vi "Entry.vi"(8 "error in (no error)":errorcluster, 11 "New State":refnum<class "Init.lvclass">) -> (0 "error out":errorcluster, 3 "State out":refnum<class "Init.lvclass">)   [LabVIEW 2024, in "Chef State.lvlib" / "Init.lvclass"]
doc: "This is an abstract method. Override this method to define the behavior when you enter the state."
uses:
  Init.lvclass
  C:/Program Files/National Instruments/LabVIEW 2024/vi.lib/ActorFramework/Actor/Actor.lvclass
  <vilib>/ActorFramework/Actor/Actor.lvclass/Actor.ctl
  Chef UI Logic/Chef UI Logic Messages/Update Log Msg/Update Log Msg.lvclass/Update Log Msg.ctl
  <vilib>/ActorFramework/Message Enqueuer/Message Enqueuer.lvclass/Message Enqueuer.ctl
  <vilib>/ActorFramework/Message Enqueuer/Enqueue.vi
  <vilib>/ActorFramework/Message Enqueuer/Init from Existing Queue.vi
  Chef UI Logic/Chef UI Logic Messages/Update Log Msg/Update Log Msg.lvclass
  C:/Program Files/National Instruments/LabVIEW 2024/vi.lib/ActorFramework/Message/Message.lvclass
  Chef State Messages/Go to Idle Msg/Go to Idle Msg.lvclass
  <vilib>/ActorFramework/Message Priority Queue/Priority Enqueue.vi
  Chef State/Chef State.lvclass
  <vilib>/ActorFramework/Message Enqueuer/Message Enqueuer.lvclass
  Init.lvclass/Init.ctl
  <vilib>/ActorFramework/Actor/Actor.lvclass
  Chef UI Messages/Go to Idle State Msg/Go to Idle State Msg.lvclass
  C:/Users/burakkorkmaz/Desktop/PROJE/actor-state-machine/Chef State/Chef State/Chef State.lvclass
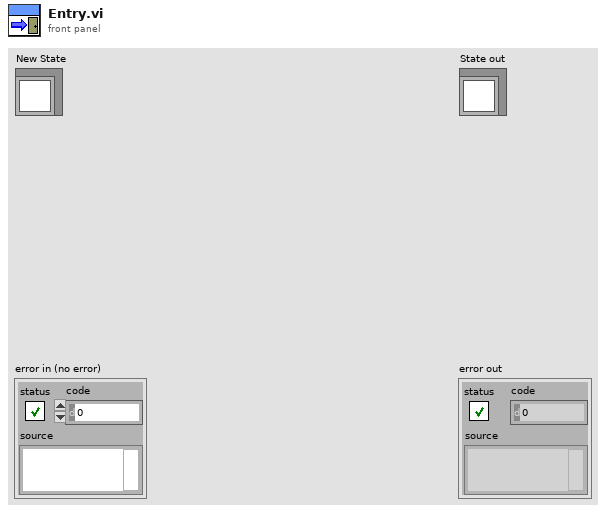
[diagram p1: front panel]
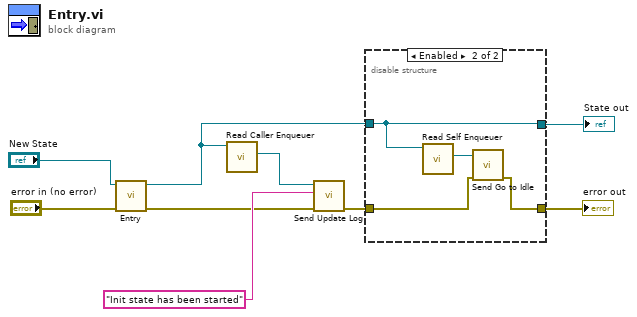
[diagram p0: block diagram]
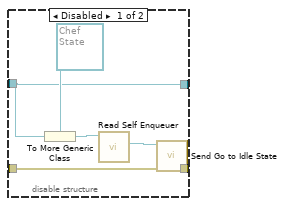
[diagram p2: hidden frame]
diagram:
  n1 = call-parent "Entry.vi"("error in (no error)"="error in (no error)", "New State"="New State") -> ("error out"=w5:errorcluster, "State out"=w2:refnum<class "Init.lvclass">)  [unwired: 8 in]
  n2 = call <vilib>:"Read Caller Enqueuer.vi"("Actor"=w2) -> ("Caller Enqueuer"=w7:refnum<class "Message Enqueuer.lvclass">)  [unwired: 10 in]
  n3 = call "Send Update Log.vi"("error in (no error)"=w5, "Log"="Init state has been started", "Message Enqueuer"=w7) -> ("error out"=w3:errorcluster)  [unwired: 7 in, 1 out]
  n4 = disable-structure shown="Enabled" {
    disable-tunnel: [w15 w16] -> w4
    disable-tunnel: w2 -> [w10 w18]
    disable-tunnel: w3 -> [w11 w17]
    disable-tunnel: [w10 w18] -> w1
    frame Disabled {
      n5 = To More Generic Class(target class=refnum<class "Chef State.lvclass"> refnum ("Chef State.lvlib:Chef State.lvclass"), reference=w10) -> (generic class reference=w13:refnum<class "Chef State.lvclass">)
      n6 = call <vilib>:"Read Self Enqueuer.vi"("Actor"=w13) -> ("Self Enqueuer"=w14:refnum<class "Message Enqueuer.lvclass">)  [unwired: 10 in]
      n7 = call "Send Go to Idle State.vi"("error in (no error)"=w11, "Message Enqueuer"=w14) -> ("error out"=w15:errorcluster)  [unwired: 8 in, 1 out]
    }
    frame Enabled {
      n8 = call <vilib>:"Read Self Enqueuer.vi"("Actor"=w18) -> ("Self Enqueuer"=w19:refnum<class "Message Enqueuer.lvclass">)  [unwired: 10 in]
      n9 = call "Send Go to Idle.vi"("error in (no error)"=w17, "Message Enqueuer"=w19) -> ("error out"=w16:errorcluster)  [unwired: 8 in, 1 out]
    }
  }
  "error out" <- w4
  "State out" <- w1
